vi "Icon.vi"(11 "Build Package Item in":refnum<class "VIPM Item.lvclass">) -> (2 "Icon":T1 caption="Icon (16x16 px)")   [LabVIEW 2019, in "VIPM.lvlib" / "VIPM Item.lvclass"]
uses:
  VIPM Item.lvclass
  libs/Solution.lvlibp/1abvi3w/vi.lib/picture/picture.llb/imagedata.ctl
  VIPM Item.lvclass/VIPM Item.ctl
  libs/Solution.lvlibp
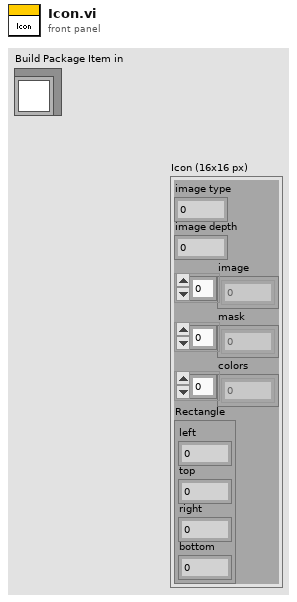
[diagram p1: front panel]
types:
  T1 = typedef "Solution.lvlibp/imagedata.ctl" = cluster{"image type":i32, "image depth":i32, "image":u8[], "mask":u8[], "colors":u32[], "Rectangle":cluster{"left":i16, "top":i16, "right":i16, "bottom":i16}}
  T2 = typedef "VIPM.lvlib/VIPM Item.lvclass/File Type.ctl" = enum16{"Unsupported", "VIPB", "VIPC"}
  T3 = cluster{"width":u32, "height":u32, "colors":u32, "color table":u32[], "data":u8[], "icon mask data":u8[]}[]
  T4 = typedef "IconInfo.ctl" = cluster{"Width":u8, "Height":u8, "Depth":u8, "Resource Data":u8[]}
  T5 = cluster{"left":i16, "top":i16, "right":i16, "bottom":i16}
  T6 = cluster{"width":u32, "height":u32, "colors":u32, "color table":u32[], "data":u8[], "icon mask data":u8[]}
  T7 = typedef "imagedata.ctl" = cluster{"image type":i32, "image depth":i32, "image":u8[], "mask":u8[], "colors":u32[], "Rectangle":cluster{"left":i16, "top":i16, "right":i16, "bottom":i16}}
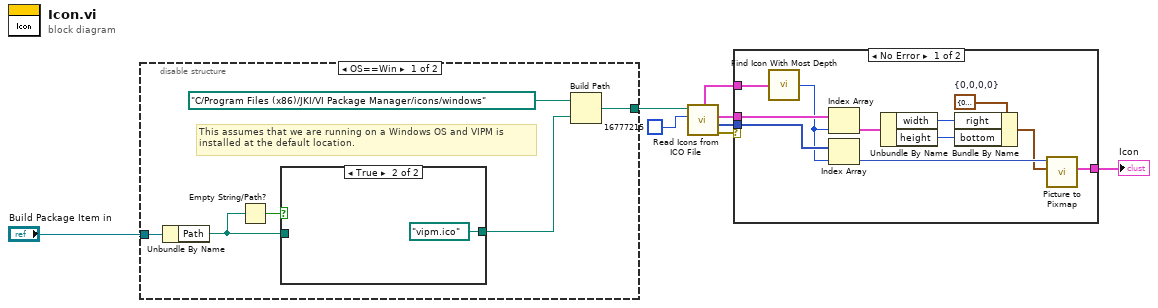
[diagram p0: block diagram]
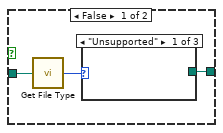
[diagram p2: hidden frame]
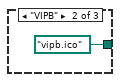
[diagram p3: hidden frame]
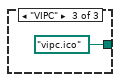
[diagram p4: hidden frame]
diagram:
  n1 = disable-structure shown="OS==Win" {
    disable-tunnel: [w11 _] -> w8
    disable-tunnel: "Build Package Item in" -> [w14 _]
    frame condition #0 (active) {
      # "This assumes that we are running on a Windows OS and VIPM is\ninstalled at the default location."
      n2 = Unbundle By Name(w14) -> ("Path"=w10:path)
      n3 = Empty String/Path?(string/path=w10) -> (empty?=w9:bool)
      n4 = case shown="True" w9 {
        tunnel: [w16 path "vipm.ico"] -> w13
        tunnel: w10 -> [w15 _]
        frame False {
          n5 = call "Get File Type.vi"("Path"=w15) -> ("File Type"=w17:T2)  [unwired: 1 in]
          n6 = case shown="\"Unsupported\"" w17 {
            tunnel: [_ path "vipb.ico" path "vipc.ico"] -> w16
            frame "Unsupported" {
            }
            frame "VIPB" {
            }
            frame "VIPC" {
            }
          }
        }
        frame True {
        }
      }
      n7 = Build Path(base path=path "C:/Program Files (x86)/JKI/VI Package Manager/icons/windows" ("path to JPEG file"), name or relative path=w13) -> (appended path=w11:path)
    }
    frame condition #1 {
    }
  }
  n8 = call <vilib>:"Read Icons from ICO File.vi"("background color(black)"=u32 16777215, "file path"=w8) -> ("error out"=w4:errorcluster, "icon pictures"=w7:picture[], "icon data"=w6:T3, "Icon Info"=w1:T4[])  [unwired: 5 in, 1 out]
  n9 = case shown="No Error" w4 {
    tunnel: w7 -> [w31 _]
    tunnel: w6 -> [w30 _]
    tunnel: [w23 _] -> w3
    tunnel: w1 -> [w22 _]
    frame No Error {
      w27 = T5 {"left"=0, "top"=0, "right"=0, "bottom"=0}  # {0,0,0,0}
      n10 = call "Find Icon With Most Depth.vi"("Icon Info"=w22) -> ("Icon Index"=w21:i32)  [unwired: 1 in]
      n11 = Index Array(array=w30, index=w21) -> (element=w29:T6)
      n12 = Index Array(array=w31, index=w21) -> (element=w28:picture)
      n13 = Unbundle By Name(w29) -> ("width"=w26:u32, "height"=w25:u32)
      n14 = Bundle By Name(cluster=w27, "right"=w26, "bottom"=w25) -> (w24:T5)
      n15 = call <vilib>:"Picture to Pixmap.vi"("rect"=w24, "picture"=w28) -> ("image data"=w23:T7)  [unwired: 8 in, 1 out]
    }
    frame Error {
    }
  }
  "Icon" <- w3
